vi "LIN EX Master Start Sch.vi"(7 "MsgLen":u32, 8 "error in (no error)":errorcluster, 9 "pLINMsg":T1, 10 "LINIndex":u8, 11 "DevHandle":i32) -> (0 "error out":errorcluster, 1 "pLINMsg out":T1, 3 "function return":i32)   [LabVIEW 2010, in "usb2lin_ex.lvlib"]
doc: "int WINAPI LIN_EX_MasterStartSch(int DevHandle,unsigned char LINIndex,LIN_EX_MSG *pLINMsg,unsigned int MsgLen);"
uses:
  usb2lin_ex.lvlib
  USB2XXX/trunk/USB2XXX/USB2XXX/vs2010/Release/USB2XXX.dll
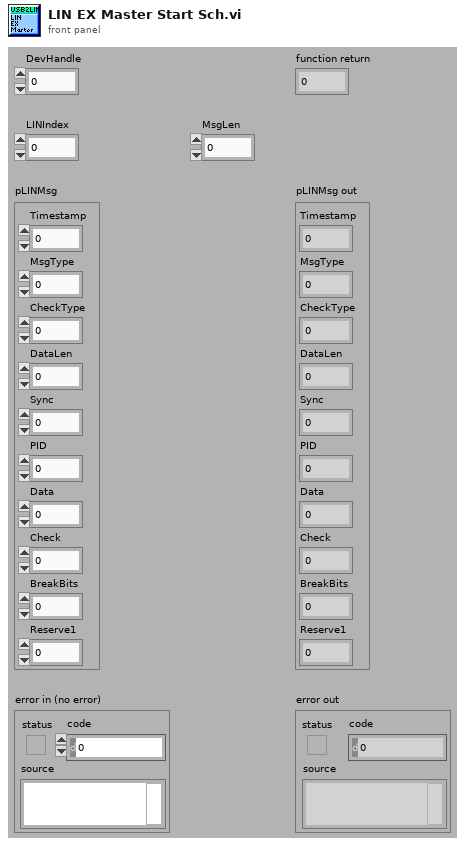
[diagram p1: front panel]
types:
  T1 = cluster{"Timestamp":u32, "MsgType":u8, "CheckType":u8, "DataLen":u8, "Sync":u8, "PID":u8, "Data":u8, "Check":u8, "BreakBits":u8, "Reserve1":u8}
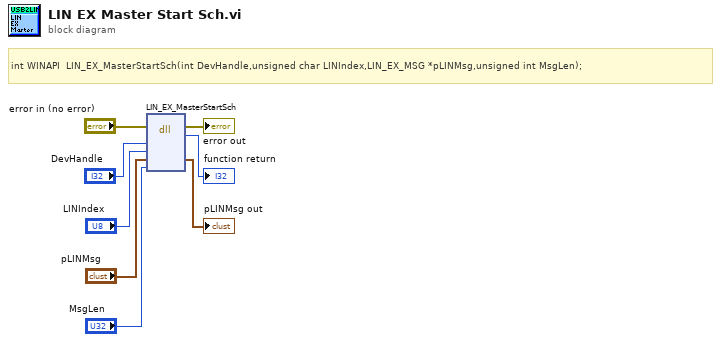
[diagram p0: block diagram]
diagram:
  # "int WINAPI  LIN_EX_MasterStartSch(int DevHandle,unsigned char LINIndex,LIN_EX_MSG *pLINMsg,unsigned int MsgLen);"
  n1 = dll-call lib="E:/OtherWork/STM32/USB2XXX/trunk/USB2XXX/USB2XXX/vs2010/Release/USB2XXX.*" fn="LIN_EX_MasterStartSch"(error in="error in (no error)", "DevHandle"="DevHandle", "LINIndex"="LINIndex", "pLINMsg"="pLINMsg", "MsgLen"="MsgLen") -> (error out=→"error out":errorcluster, →"function return":i32, "pLINMsg"=→"pLINMsg out":T1)  [unwired: 5 in, 1 out]
